vi "Instr_SetPrivateData.vi"(8 "error in (no error)":errorcluster, 11 "WK6440B in":refnum<class "WK6440B.lvclass">) -> (0 "error out":errorcluster, 3 "WK6440B out":refnum<class "WK6440B.lvclass">)   [LabVIEW 2013, in "WK6440B.lvclass"]
uses:
  WK6440B.lvclass
  InstrumentSetup.vi
  WK6440B_CommandsGlobal.vi
  InstrControl.lvclass
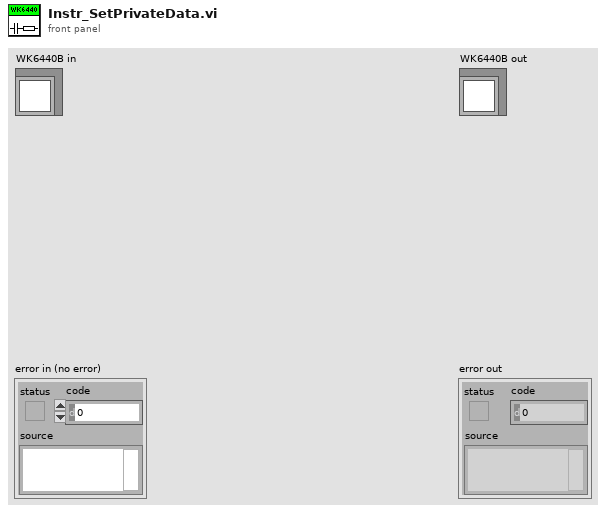
[diagram p1: front panel]
types:
  T1 = cluster{"RC Configuration":u16, "AC amplitude [V]":dbl, "AC frequency [Hz]":i32, "GPIB Address":string}
  T2 = cluster{"GPIB address":string, "Instrument name":string, "Instrument type":u16, "Command \"Initialise LCR\"":string, "Command \"OC Trim\"":string, "Command \"LCR Readout\"":string}
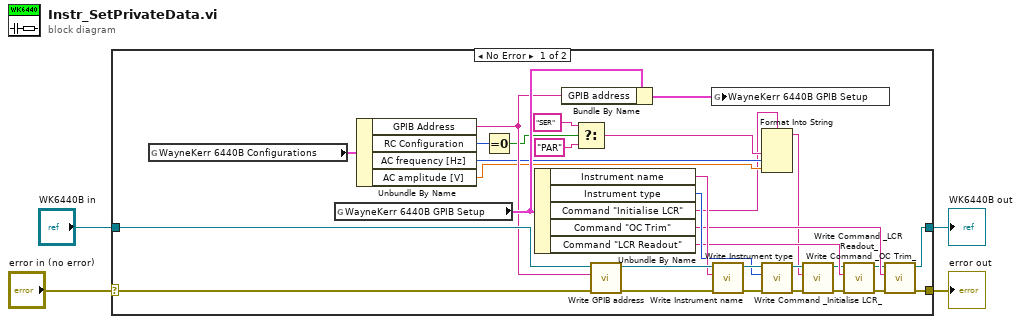
[diagram p0: block diagram]
diagram:
  n1 = case shown="No Error" "error in (no error)" {
    selector: "error in (no error)" -> [w30 w37]
    tunnel: [w17 w37] -> w3
    tunnel: [w18 w36] -> w1
    tunnel: "WK6440B in" -> [w35 w36]
    frame No Error {
      n2 = global read "InstrumentSetup.vi" "WayneKerr 6440B Configurations"() -> (w27:T1)
      n3 = global read "WK6440B_CommandsGlobal.vi" "WayneKerr 6440B GPIB Setup"() -> (w25:T2)
      n4 = Unbundle By Name(w27) -> ("GPIB Address"=w24:string, "RC Configuration"=w13:u16, "AC frequency [Hz]"=w8:i32, "AC amplitude [V]"=w7:dbl)
      n5 = Equal To 0?(x=w13) -> (x = 0?=w12:bool)
      n6 = Unbundle By Name(w25) -> ("Instrument name"=w32:string, "Instrument type"=w31:u16, "Command \"Initialise LCR\""=w6:string, "Command \"OC Trim\""=w22:string, "Command \"LCR Readout\""=w23:string)
      n7 = Bundle By Name(cluster=w25, "GPIB address"=w24) -> (w26:T2)
      n8 = Select(t="SER", s=w12, f="PAR") -> (s? t:f=w9:string)
      n9 = call-dynamic "Write GPIB address.vi"("error in (no error)"=w30, "GPIB address"=w24, "InstControl in"=w35) -> ("error out"=w29:errorcluster, "InstControl out"=w34:refnum<class "WK6440B.lvclass">)  [unwired: 7 in]
      n10 = global write "WK6440B_CommandsGlobal.vi" "WayneKerr 6440B GPIB Setup"(w26) -> ()
      n11 = call-dynamic "Write Instrument name.vi"("error in (no error)"=w29, "Instrument name"=w32, "InstControl in"=w34) -> ("error out"=w28:errorcluster, "InstControl out"=w33:refnum<class "WK6440B.lvclass">)  [unwired: 7 in]
      n12 = Format Into String(format string=w6, w9, w8, w7) -> (resulting string=w5:string)  [unwired: 2 in, 1 out]
      n13 = call-dynamic "Write Instrument type.vi"("error in (no error)"=w28, "Instrument type"=w31, "InstControl in"=w33) -> ("error out"=w14:errorcluster, "InstControl out"=w21:refnum<class "WK6440B.lvclass">)  [unwired: 7 in]
      n14 = call-dynamic "Write Command _Initialise LCR_.vi"("error in (no error)"=w14, "Command \"Initialise LCR\""=w5, "LCRControl in"=w21) -> ("error out"=w16:errorcluster, "LCRControl out"=w20:refnum<class "WK6440B.lvclass">)  [unwired: 7 in]
      n15 = call-dynamic "Write Command _LCR Readout_.vi"("error in (no error)"=w16, "Command \"LCR Readout\""=w23, "LCRControl in"=w20) -> ("error out"=w15:errorcluster, "LCRControl out"=w19:refnum<class "WK6440B.lvclass">)  [unwired: 7 in]
      n16 = call-dynamic "Write Command _OC Trim_.vi"("error in (no error)"=w15, "Command \"OC Trim\""=w22, "LCRControl in"=w19) -> ("error out"=w17:errorcluster, "LCRControl out"=w18:refnum<class "WK6440B.lvclass">)  [unwired: 7 in]
    }
    frame Error {
    }
  }
  "error out" <- w3
  "WK6440B out" <- w1
